vi "DAQ- Steper.vi"(0 "Travel (Degree)":dbl=100.0, 1 "Mode":i32(ring)=10178 items=["Finite Samples"=10178, "Continuous Samples"=10123, "Hardware Timed Single Point"=12522], 5 "Home Condition":bool, 7 "Speed d/s":dbl=10.0, 11 "error in":errorcluster) -> (4 "Task Done Bit":bool, 14 "error out":errorcluster)   [LabVIEW 2015]
uses:
  Project Setup/Globle Variable/GR_Servo.vi
  Galobal variable_TI.vi
  <vilib>/DAQmx/create/channels.llb/DAQmx Create Channel (CO-Pulse Generation-Frequency).vi
  <vilib>/DAQmx/configure/timing.llb/DAQmx Timing (Implicit).vi
panel:
  in  "Motor PPR":dbl=3600.0
  in  "Motor Gear Ratio":dbl=1.0
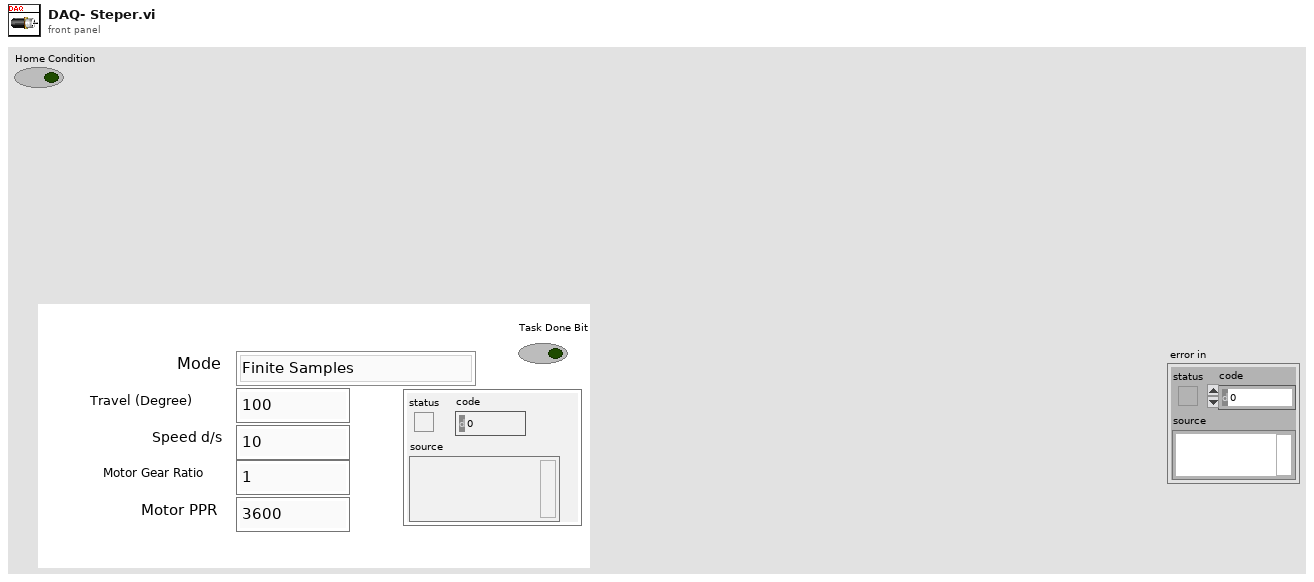
[diagram p1: front panel]
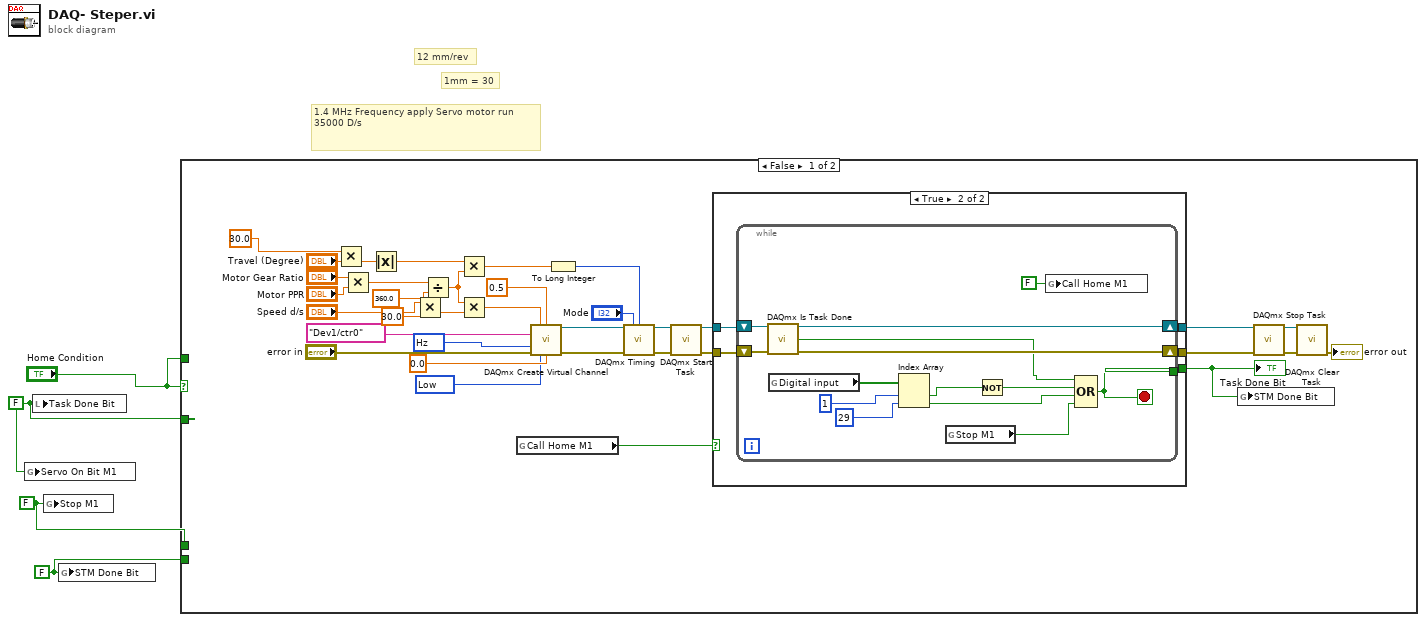
[diagram p0: block diagram]
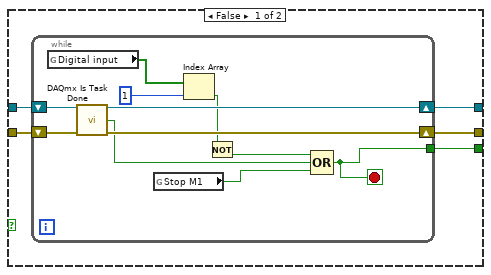
[diagram p2: hidden frame]
diagram:
  w1 = FALSE ("STM Done Bit")
  w3 = FALSE ("Stop M1")
  w4 = FALSE ("Task Done Bit")
  # "1mm = 30"
  # "12 mm/rev"
  # "1.4 MHz Frequency apply Servo motor run \n35000 D/s"
  n1 = global write "GR_Servo.vi" "Servo On Bit M1"(w4) -> ()
  n2 = local write "Task Done Bit"(w4) -> ()
  n3 = global write "Galobal variable_TI.vi" "Stop M1"(w3) -> ()
  n4 = global write "Galobal variable_TI.vi" "STM Done Bit"(w1) -> ()
  n5 = case shown="False" "Home Condition" {
    tunnel: w4 -> [_ _]
    tunnel: w3 -> [_ _]
    tunnel: "Home Condition" -> [_ _]
    tunnel: w1 -> [_ _]
    frame False {
      w15 = 10373 items=["Hz"=10373] ("units")
      w16 = 10214 items=["High"=10192, "Low"=10214] ("idle state")
      n6 = Multiply(x=30.0, y="Travel (Degree)") -> (x*y=w11:dbl)
      n7 = Multiply(x="Motor Gear Ratio", y="Motor PPR") -> (x*y=w25:dbl)
      n8 = Absolute Value(x=w11) -> (abs(x)=w24:dbl)
      n9 = Multiply(x="Speed d/s", y=30.0) -> (x*y=w9:dbl)
      n10 = Divide(x=w25, y=360.0) -> (x/y=w31:dbl)
      n11 = Multiply(x=w24, y=w31) -> (x*y=w29:dbl)
      n12 = Multiply(x=w31, y=w9) -> (x*y=w36:dbl)
      n13 = global read "Galobal variable_TI.vi" "Call Home M1"() -> (w6:bool)
      n14 = call-poly <vilib>:"DAQmx Create Virtual Channel.vi"("frequency"=w36, "duty cycle"=0.5, "counter"=tag "Dev1/ctr0", "units"=w15, "error in"="error in", "idle state"=w16, "initial delay"=0.0) -> ("task out"=w18:refnum<k21>, "error out"=w19:errorcluster)  [unwired: 7 in]
      n15 = To Long Integer(number=w29) -> (32bit integer=w39:i32)
      n16 = call-poly <vilib>:"DAQmx Timing.vi"("task/channels in"=w18, "sample mode"="Mode", "samples per channel"=w39, "error in"=w19) -> ("task out"=w20:refnum<k21>, "error out"=w21:errorcluster)  [unwired: 10 in]
      n17 = call <vilib>:"DAQmx Start Task.vi"("task/channels in"=w20, "error in"=w21) -> ("task out"=w14:refnum<k21>, "error out"=w12:errorcluster)  [unwired: 12 in]
      n18 = case shown="True" w6 {
        tunnel: [w44 w57] -> w34
        tunnel: w14 -> [w43 w60]
        tunnel: [w42 w58] -> w13
        tunnel: w12 -> [w41 w59]
        tunnel: [w40 w56] -> w5
        frame False {
          n19 = while {
            shift-right: [w53] -> w42
            shift-left: w43 -> [w55]
            shift-right: [w54] -> w44
            shift-left: w41 -> [w52]
            tunnel: [w51] -> w40
            stop <- w51 stop-if-true
            n20 = global read "Galobal variable_TI.vi" "Digital input"() -> (w50:bool[])
            n21 = call <vilib>:"DAQmx Is Task Done.vi"("task/channels in"=w55, "error in"=w52) -> ("task out"=w53:refnum<k21>, "task done?"=w47:bool, "error out"=w54:errorcluster)  [unwired: 11 in]
            n22 = global read "Galobal variable_TI.vi" "Stop M1"() -> (w48:bool)
            n23 = Index Array(array=w50, index=1) -> (element=w46:bool)
            n24 = Not(x=w46) -> (.not. x?=w45:bool)
            n25 = Compound Arithmetic op=OR(w45, w47, w48) -> (w51:bool)
          }
        }
        frame True {
          n26 = while {
            shift-right: [w72] -> w58
            shift-left: w60 -> [w74]
            shift-right: [w73] -> w57
            shift-left: w59 -> [w71]
            tunnel: [w67] -> w56
            stop <- w67 stop-if-true
            n27 = call <vilib>:"DAQmx Is Task Done.vi"("task/channels in"=w74, "error in"=w71) -> ("task out"=w72:refnum<k21>, "task done?"=w64:bool, "error out"=w73:errorcluster)  [unwired: 11 in]
            n28 = global read "Galobal variable_TI.vi" "Digital input"() -> (w68:bool[])
            n29 = Index Array(array=w68, index #1=1 ("index"), index #2=29 ("index")) -> (element #1=w63:bool, element #2=w62:bool)
            n30 = global read "Galobal variable_TI.vi" "Stop M1"() -> (w70:bool)
            n31 = Not(x=w63) -> (.not. x?=w61:bool)
            n32 = global write "Galobal variable_TI.vi" "Call Home M1"(FALSE ("Call Home M1")) -> ()
            n33 = Compound Arithmetic op=OR(w64, w61, w62, w70) -> (w67:bool)
          }
        }
      }
      "Task Done Bit" <- w5
      n34 = global write "Galobal variable_TI.vi" "STM Done Bit"(w5) -> ()
      n35 = call <vilib>:"DAQmx Stop Task.vi"("task/channels in"=w13, "error in"=w34) -> ("task out"=w22:refnum<k21>, "error out"=w35:errorcluster)  [unwired: 12 in]
      n36 = call <vilib>:"DAQmx Clear Task.vi"("task in"=w22, "error in"=w35) -> ("error out"=→"error out":errorcluster)  [unwired: 13 in]
    }
    frame True {
    }
  }
